vi "Set Progress WD.vi"(8 "error in (no error)":errorcluster, 10 "Progress WD":refnum<user-event>, 11 "Search in":refnum<class "Search.lvclass">) -> (0 "error out":errorcluster, 3 "Search out":refnum<class "Search.lvclass">)   [LabVIEW 2016, in "Better Search.lvlib" / "Search.lvclass"]
uses:
  Search.lvclass
  Search Progress.ctl
  Better Search.lvlib
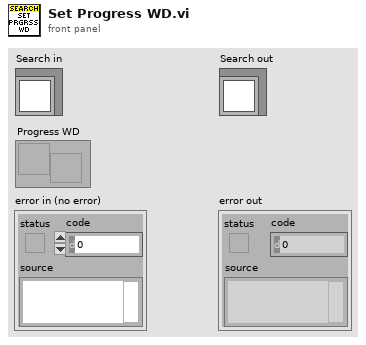
[diagram p1: front panel]
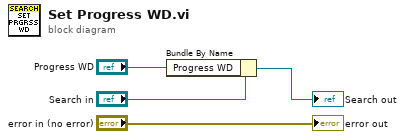
[diagram p0: block diagram]
diagram:
  n1 = Bundle By Name(cluster="Search in", "Progress WD"="Progress WD") -> (→"Search out":refnum<class "Search.lvclass">)
  "error out" <- "error in (no error)"
